vi "Get Owner.vi"(8 "error in (no error)":errorcluster, 11 "ArrayPanel in":refnum<class "ArrayPanel.lvclass">) -> (0 "error out":errorcluster, 2 "Owner":refnum<class "ArrayManager.lvclass">, 3 "ArrayPanel out":refnum<class "ArrayPanel.lvclass">)   [LabVIEW 2014, in "OOPanel.lvlib" / "ArrayPanel.lvclass"]
uses:
  ArrayPanel.lvclass
  ArrayManager/ArrayManager.lvclass
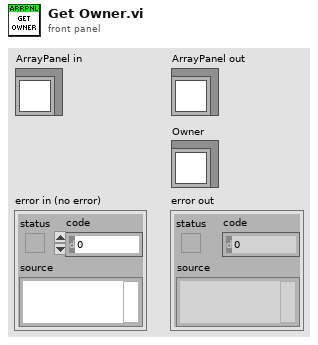
[diagram p1: front panel]
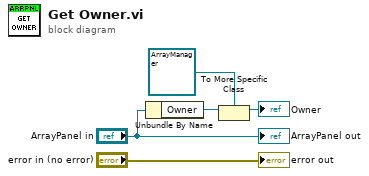
[diagram p0: block diagram]
diagram:
  n1 = Unbundle By Name("ArrayPanel in") -> ("Owner"=w3:refnum<class>)
  n2 = To More Specific Class(target class=refnum<class "ArrayManager.lvclass"> refnum ("OOPanel.lvlib:ArrayManager.lvclass"), reference=w3) -> (specific class reference=→"Owner":refnum<class "ArrayManager.lvclass">)  [unwired: 1 in, 1 out]
  "error out" <- "error in (no error)"
  "ArrayPanel out" <- "ArrayPanel in"
